vi "cluster_v02.vi"() -> ()   [LabVIEW 2009]
panel:
  in  "stop":bool
  in  "x_max":i32(knob)=6 scale=0.0..10.0
  out "x":dbl=5.999999999999968
  out "Graficul functiei e^x":cluster{dbl[], dbl[]}(graph)
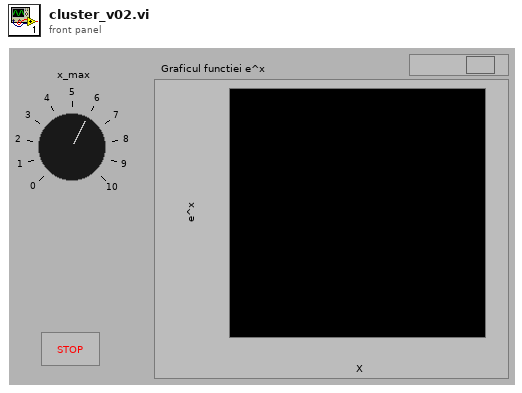
[diagram p1: front panel]
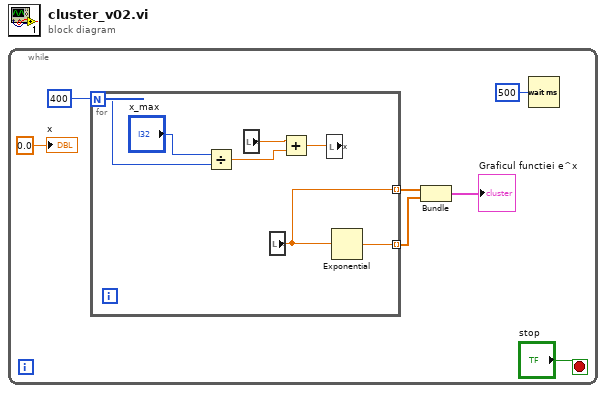
[diagram p0: block diagram]
diagram:
  n1 = while {
    stop <- "stop" stop-if-true
    n2 = for {
      N: 400 -> [w10]
      tunnel: [w9] -> w6 mode=indexing
      tunnel: [w14] -> w5 mode=indexing
      n3 = Divide(x="x_max", y=w10) -> (x/y=w11:dbl)
      n4 = local read "x"() -> (w12:dbl)
      n5 = local read "x"() -> (w9:dbl)
      n6 = Add(x=w12, y=w11) -> (x+y=w13:dbl)
      n7 = local write "x"(w13) -> ()
      n8 = Exponential(1:w9) -> (0:w14:dbl)
    }
    n9 = Bundle(w6, w5) -> (→"Graficul functiei e^x":cluster{dbl[], dbl[]})  [unwired: 1 in]
    n10 = Wait (ms)(milliseconds to wait=u32 500) -> ()  [unwired: 1 out]
    "x" <- 0.0 ("x")
  }
